vi "ECE3709L_Final_Project_Lab11.vi"() -> ()   [LabVIEW 2025]
uses:
  <vilib>/Instr/_visa.llb/VISA Configure Serial Port (Instr).vi
panel:
  in  "VISA resource name":refnum<visa-resource-name>
  out "Motor Status":string
  out "Error Message":string
  out "System Status":string
  out "Light Level (%)":dbl format="%#_1f"
  out "Humidity (%)":dbl format="%#_1f"
  out "Temperature (F)":dbl format="%#_1f"
  out "Motor RPM":dbl format="%#_1f"
  out "Mode":string
  in  "PID Enable":bool
  in  "Setpoint (RPM)":dbl format="%#_1f"
  out "Connected":bool
  in  "BAUDE RATE":dbl
  in  "Stop Program":bool
  in  "Stop":bool
  in  "Reverse":bool
  in  "Forward":bool
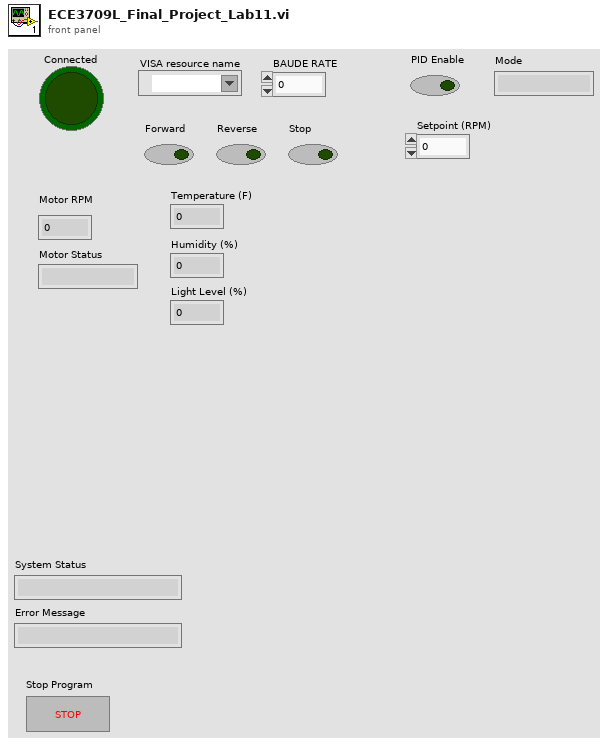
[diagram p1: front panel]
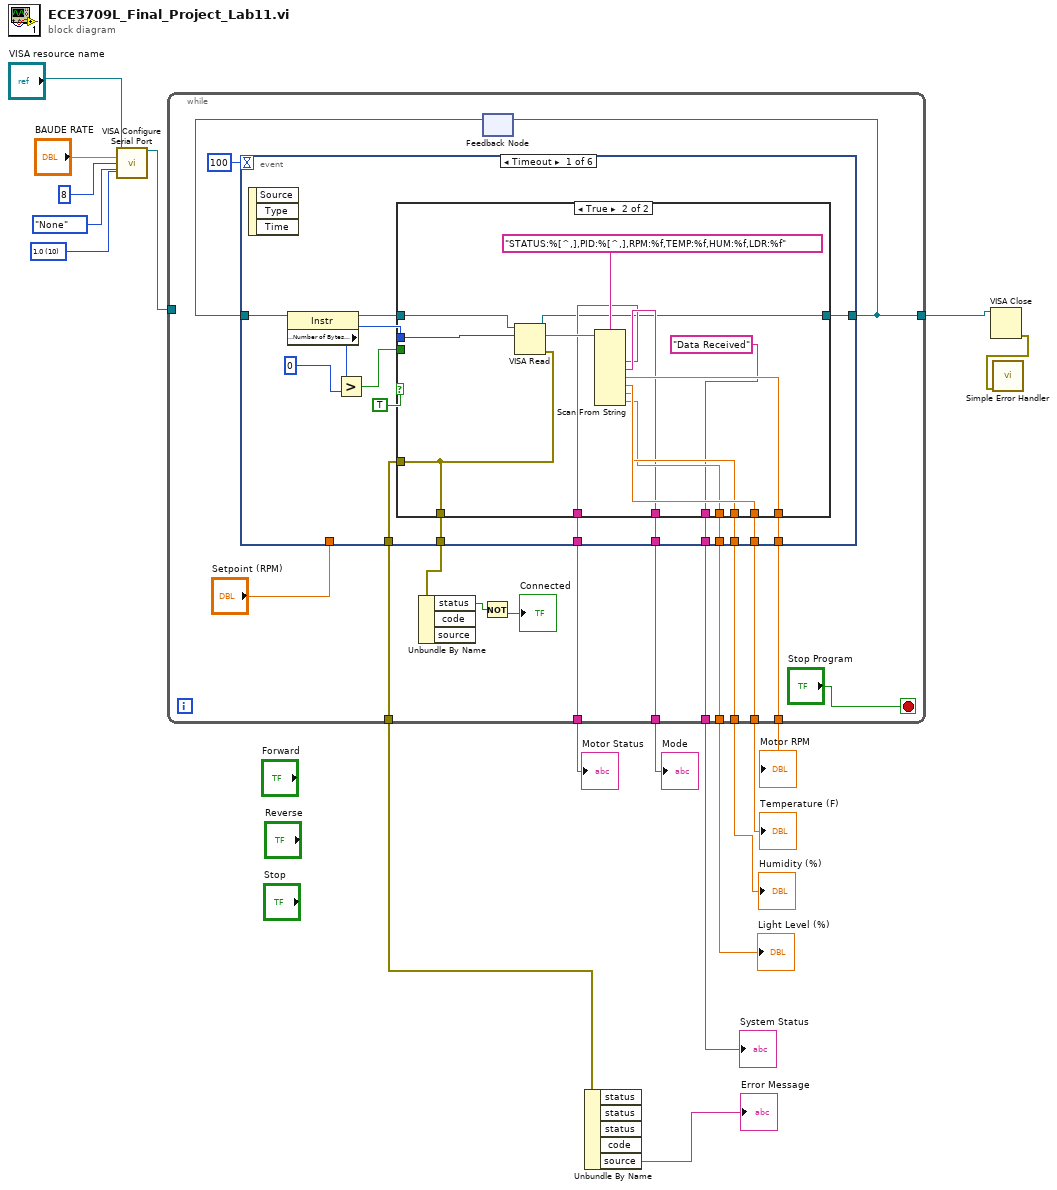
[diagram p0: block diagram]
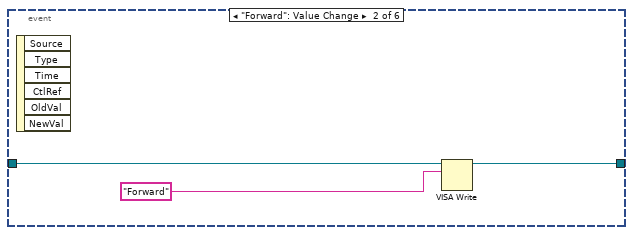
[diagram p3: hidden frame]
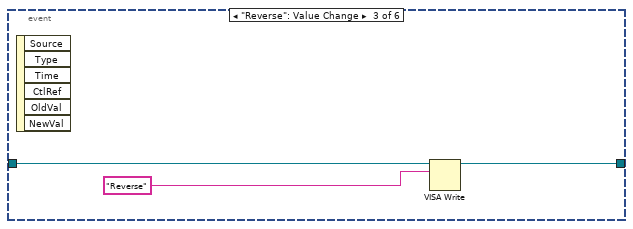
[diagram p4: hidden frame]
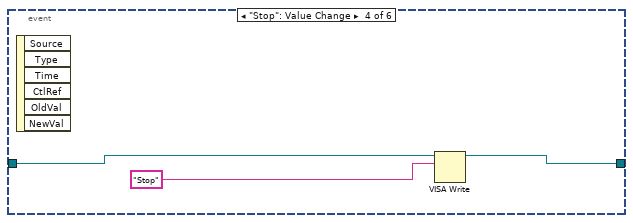
[diagram p5: hidden frame]
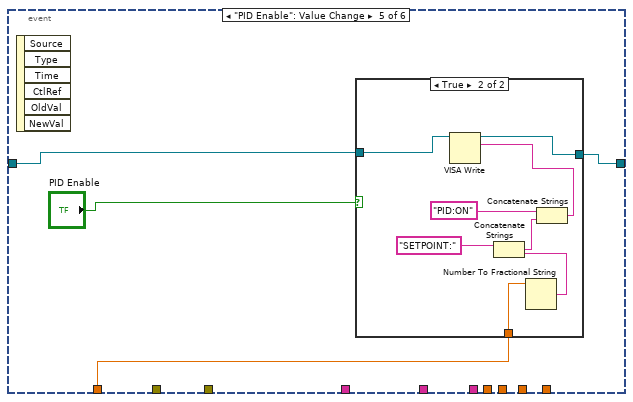
[diagram p6: hidden frame]
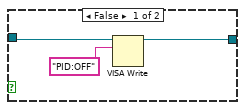
[diagram p7: hidden frame]
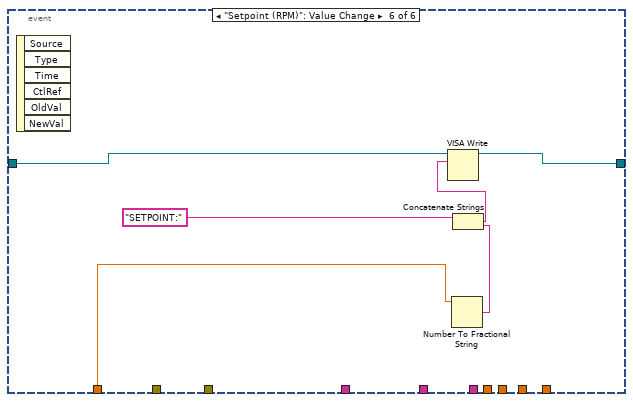
[diagram p8: hidden frame]
diagram:
  w14 = u16 10 items=["1.0"=10, "1.5"=15, "2.0"=20] ("stop bits (10: 1 bit)")
  n1 = call-poly "VISA Configure Serial Port"("VISA resource name"="VISA resource name", "baud rate (9600)"="BAUDE RATE", "data bits (8)"=u16 8, "parity (0:none)"=enum16{"None", "Odd", "Even", "Mark", "Space"}."None", "stop bits (10: 1 bit)"=w14) -> ("VISA resource name out"=w5:refnum<visa-resource-name>)  [unwired: 9 in, 1 out]
  n2 = while {
    tunnel: [w30] -> w13
    tunnel: [w29] -> w12
    tunnel: [w28] -> w11
    tunnel: [w27] -> w10
    tunnel: [w26] -> w9
    tunnel: [w25] -> w8
    tunnel: [w23] -> w7
    tunnel: w5 -> [_]
    tunnel: [w19] -> w4
    tunnel: [w18] -> w3
    stop <- "Stop Program" stop-if-true
    n3 = feedback #1() -> (w24:refnum<visa-resource-name>)  [unwired: 1 in]
    n4 = event shown="[0] Timeout" {
      selector: _ -> [_ _ _ _ _ _]
      dyn-events: _ -> [_ _ _ _ _ _]
      timeout: 100 -> [_ _ _ _ _ _]
      tunnel: w24 -> [w49 w65 w68 w71 w75 w89]
      tunnel: [w39 w64 w67 w70 w74 w88] -> w23
      tunnel: "Setpoint (RPM)" -> [_ _ _ _ w73 w92]
      tunnel: [w45 _ _ _ _ _] -> w30
      tunnel: [w44 _ _ _ _ _] -> w29
      tunnel: [w43 _ _ _ _ _] -> w28
      tunnel: [w42 _ _ _ _ _] -> w27
      tunnel: [w41 _ _ _ _ _] -> w26
      tunnel: [w40 _ _ _ _ _] -> w25
      tunnel: [w38 _ _ _ _ _] -> w22
      tunnel: [w37 _ _ _ _ _] -> w19
      tunnel: [w36 _ _ _ _ _] -> w18
      event Timeout {
        n5 = event-data() -> ()  [unwired: 1 in, 3 out]
        n6 = property class="Instr"(reference=w49) -> (reference out=w46:refnum<visa-resource-name>, "Serial Settings:Number of Bytes at Serial Port"=w47:u32)  [unwired: 1 in, 1 out]
        n7 = Greater?(x=w47, y=u32 0) -> (0:w35:bool)
        n8 = case shown="True" TRUE {
          tunnel: w35 -> [_ _]
          tunnel: w47 -> [_ w63]
          tunnel: w46 -> [w50 w62]
          tunnel: [_ w59] -> w45
          tunnel: [_ w58] -> w44
          tunnel: [_ w57] -> w43
          tunnel: [_ w56] -> w42
          tunnel: [_ w55] -> w41
          tunnel: [_ w54] -> w40
          tunnel: [w50 w53] -> w39
          tunnel: [_ w51] -> w38
          tunnel: [_ "Data Received"] -> w37
          tunnel: [_ w51] -> w36
          frame False {
          }
          frame True {
            n9 = VISA Read(VISA resource name=w62, byte count=w63) -> (VISA resource name out=w53:refnum<visa-resource-name>, read buffer=w61:string, error out=w51:errorcluster)  [unwired: 1 in, 1 out]
            n10 = Scan From String(format string="STATUS:%[^,],PID:%[^,],RPM:%f,TEMP:%f,HUM:%f,LDR:%f", input string=w61) -> (output 1=w54:string, output 2=w55:string, output 3=w59:dbl, output 4=w58:dbl, output 5=w57:dbl, output 6=w56:dbl)  [unwired: 8 in, 3 out]
          }
        }
      }
      event "Forward": Value Change {
        n11 = event-data() -> ()  [unwired: 1 in, 6 out]
        n12 = VISA Write(VISA resource name=w65, write buffer="Forward") -> (VISA resource name out=w64:refnum<visa-resource-name>)  [unwired: 1 in, 2 out]
      }
      event "Reverse": Value Change {
        n13 = event-data() -> ()  [unwired: 1 in, 6 out]
        n14 = VISA Write(VISA resource name=w68, write buffer="Reverse") -> (VISA resource name out=w67:refnum<visa-resource-name>)  [unwired: 1 in, 2 out]
      }
      event "Stop": Value Change {
        n15 = event-data() -> ()  [unwired: 1 in, 6 out]
        n16 = VISA Write(VISA resource name=w71, write buffer="Stop") -> (VISA resource name out=w70:refnum<visa-resource-name>)  [unwired: 1 in, 2 out]
      }
      event "PID Enable": Value Change {
        n17 = event-data() -> ()  [unwired: 1 in, 6 out]
        n18 = case shown="True" "PID Enable" {
          tunnel: w75 -> [w78 w82]
          tunnel: [w77 w81] -> w74
          tunnel: w73 -> [_ w80]
          frame False {
            n19 = VISA Write(VISA resource name=w78, write buffer="PID:OFF") -> (VISA resource name out=w77:refnum<visa-resource-name>)  [unwired: 1 in, 2 out]
          }
          frame True {
            n20 = Number To Fractional String(number=w80) -> (F-format string=w85:string)  [unwired: 3 in]
            n21 = Concatenate Strings("SETPOINT:" ("string"), w85) -> (w84:string)
            n22 = Concatenate Strings("PID:ON" ("string"), w84) -> (w83:string)
            n23 = VISA Write(VISA resource name=w82, write buffer=w83) -> (VISA resource name out=w81:refnum<visa-resource-name>)  [unwired: 1 in, 2 out]
          }
        }
      }
      event "Setpoint (RPM)": Value Change {
        n24 = event-data() -> ()  [unwired: 1 in, 6 out]
        n25 = Number To Fractional String(number=w92) -> (F-format string=w91:string)  [unwired: 3 in]
        n26 = Concatenate Strings("SETPOINT:" ("string"), w91) -> (w90:string)
        n27 = VISA Write(VISA resource name=w89, write buffer=w90) -> (VISA resource name out=w88:refnum<visa-resource-name>)  [unwired: 1 in, 2 out]
      }
    }
    n28 = Unbundle By Name(w22) -> ("status"=w20:bool)  [unwired: 2 out]
    n29 = Not(x=w20) -> (.not. x?=→"Connected":bool)
    n30 = feedback-in #1(w23) -> ()
  }
  "Mode" <- w9
  "Motor RPM" <- w13
  "Temperature (F)" <- w12
  "Humidity (%)" <- w11
  "Light Level (%)" <- w10
  "System Status" <- w4
  "Motor Status" <- w8
  n31 = Unbundle By Name(w3) -> ("source"=→"Error Message":string)  [unwired: 4 out]
  n32 = VISA Close(VISA resource name=w7) -> (error out=w6:errorcluster)  [unwired: 1 in]
  n33 = call <vilib>:"Simple Error Handler.vi"("error in (no error)"=w6) -> ()  [unwired: 4 in, 5 out]
